vi "Check Subset.vi"(7 "source vi name":string, 8 "error in (no error)":errorcluster, 9 "offset (0)":u64 format="%08x bytes", 10 "length":u64 format="%08x bytes", 11 "Pointer in":refnum<class "Pointer.lvclass">) -> (0 "error out":errorcluster, 1 "offset out":u64 format="%08x bytes", 2 "length":u64 format="%08x bytes", 3 "Pointer out":refnum<class "Pointer.lvclass">)   [LabVIEW 2017, in "Memory Manager.lvlib" / "Pointer.lvclass"]
uses:
  Pointer.lvclass
  Error VIs/Out of Bounds.vi
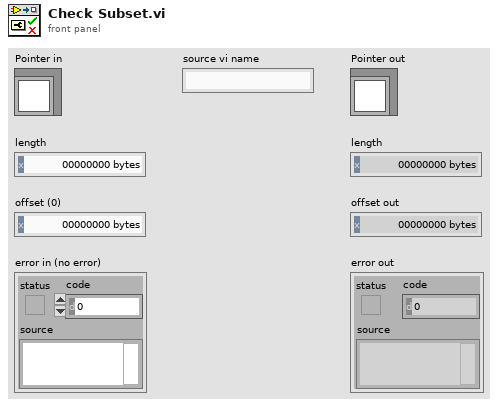
[diagram p1: front panel]
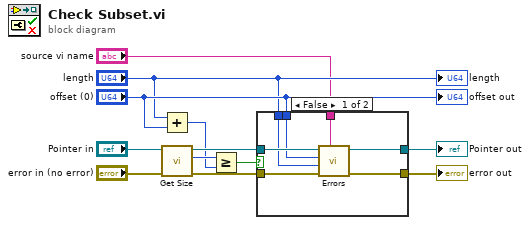
[diagram p0: block diagram]
diagram:
  n1 = Add(x="length", y="offset (0)") -> (x+y=w2:u64)
  n2 = call "Get Size.vi"("Pointer in"="Pointer in") -> ("size"=w9:u64, "Pointer out"=w4:refnum<class "Pointer.lvclass">)  [unwired: 9 in]
  n3 = Greater Or Equal?(x=w9, y=w2) -> (x >= y?=w7:bool)
  n4 = case shown="False" w7 {
    tunnel: w4 -> [w18 w19]
    tunnel: "error in (no error)" -> [w16 w20]
    tunnel: [w15 w20] -> w11
    tunnel: [w17 w19] -> w10
    tunnel: "offset (0)" -> [w14 _]
    tunnel: "length" -> [w13 _]
    tunnel: "source vi name" -> [w12 _]
    frame False {
      n5 = call-poly "Errors.vi"("error source vi name"=w12, "error in (no error)"=w16, "length"=w13, "offset"=w14, "Pointer in"=w18) -> ("error out"=w15:errorcluster, "Pointer out"=w17:refnum<class "Pointer.lvclass">)  [unwired: 5 in]
    }
    frame True {
    }
  }
  "error out" <- w11
  "Pointer out" <- w10
  "offset out" <- "offset (0)"
  "length" <- "length"
